vi "Test Project Produces Suite for Project and Nested Suite for TC.vi"(8 "error in (no error)":errorcluster, 11 "Test Case In":refnum<class "Test FInder Test.lvclass">) -> (0 "error out":errorcluster, 3 "Test Case Out":refnum<class "Test FInder Test.lvclass">)   [LabVIEW 2020, in "Test FInder Test.lvclass"]
uses:
  Test FInder Test.lvclass
  C:/Program Files (x86)/National Instruments/LabVIEW 2020/vi.lib/Astemes/LUnit/Test Case.lvclass
  source/Core/Result/Type.ctl
  <vilib>/Astemes/LUnit/Test Case.lvclass/Test Case.ctl
  4ee1ff36-f2a2-4d81-80da-2416f687ba87.vi
  <vilib>/Astemes/LUnit/Append Pass Result.vi
  <vilib>/Astemes/LUnit/Append Fail Result.vi
  <vilib>/Astemes/LUnit/Describe Comparison.vi
  <vilib>/Astemes/LUnit/Compare Variants.vi
  <vilib>/Astemes/LUnit/Variant to string.vi
  source/API/LUnit Test Suite/LUnit Test Suite.lvclass
  C:/git/astemes-lunit/source/Core/Runnable/Runnable.lvclass
  <vilib>/Utility/Data Type/Get Type Information.vi
  <vilib>/Utility/LVClass/Get LV Class Name.vi
  Test FInder Test.lvclass/Test FInder Test.ctl
  source/Framework/Test Finder/Test Finder.lvclass
  source/Core/Result/Result.lvlib
  source/Core/Runnable/Runnable.lvclass
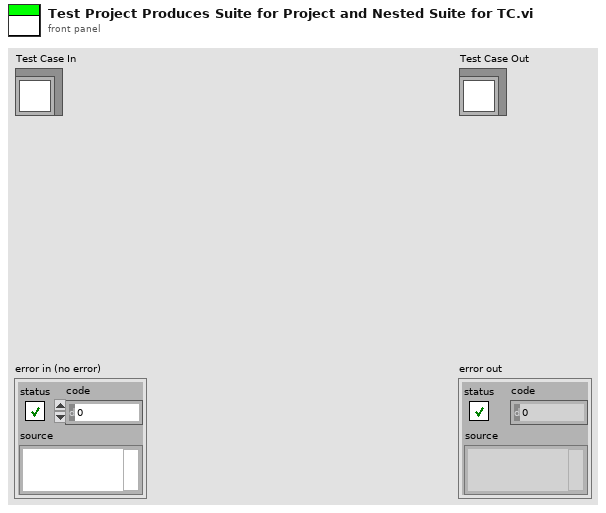
[diagram p1: front panel]
types:
  T1 = typedef "Result.lvlib/Result.ctl" = cluster{"Name":string, "Message":string, "Description":string, "Status":T2, "Result Type":T3, "Execution Time":dbl}
  T2 = typedef "Result.lvlib/Status.ctl" = enum16{"", "Passed", "Failed", "Error", "Skipped", "Setup Error", "Broken", "Teardown Error"}
  T3 = typedef "Result.lvlib/Type.ctl" = enum16{"Test Case", "Test Suite", "Test Run", "Pass", "Fail", "Skip", "Pass if", "Fail if", "Pass if Error", "Fail if Error", "Pass if Equal", "Fail if Equal"}
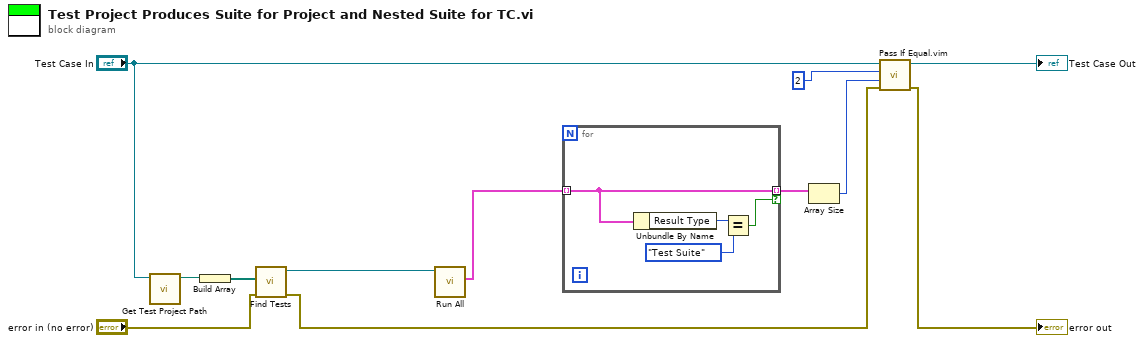
[diagram p0: block diagram]
diagram:
  n1 = call "Get Test Project Path.vi"("LUnit Test Suite Tests in"="Test Case In") -> ("appended path"=w9:path)  [unwired: 10 in]
  n2 = Build Array(w9) -> (w8:path[])
  n3 = call "Find Tests.vi"("error in (no error)"="error in (no error)", "File Paths"=w8) -> ("error out"=w10:errorcluster, "LUnit Test Suite"=w7:refnum<class "LUnit Test Suite.lvclass">)  [unwired: 8 in]
  n4 = call "Run All.vi"("Runnable In"=w7) -> ("Results"=w3:T1[])  [unwired: 9 in, 1 out]
  n5 = for {
    tunnel: w3 -> [w14] mode=indexing
    tunnel: [w14] -> w4 mode=indexing if=w13
    n6 = Unbundle By Name(w14) -> ("Result Type"=w16:T3)
    n7 = Equal?(x=w16, y=Type."Test Suite") -> (x = y?=w13:bool)
  }
  n8 = Array Size(array=w4) -> (size(s)=w2:i32)
  n9 = call "Pass If Equal.vim"("error in (no error)"=w10, "Actual"=w2, "Expected"=2 ("size(s)"), "LUnit Test Case In"="Test Case In") -> ("error out"=→"error out":errorcluster, "LUnit Test Case Out"=→"Test Case Out":refnum<class "Test FInder Test.lvclass">)  [unwired: 6 in]
